vi "getAllChannelNames.vi"(8 "error in (no error)":errorcluster, 11 "ChannelArray in":refnum<class "ChannelArray.lvclass">) -> (0 "error out":errorcluster, 2 "channelNames":string[](array[string]), 3 "ChannelArray out":refnum<class "ChannelArray.lvclass">)   [LabVIEW 2009, in "Tools.lvlib" / "DatabaseHelpers.lvlib" / "ChannelArray.lvclass"]
uses:
  ChannelArray.lvclass
  ChannelArray.lvclass/ChannelArray.ctl
  Channel/Channel.lvclass
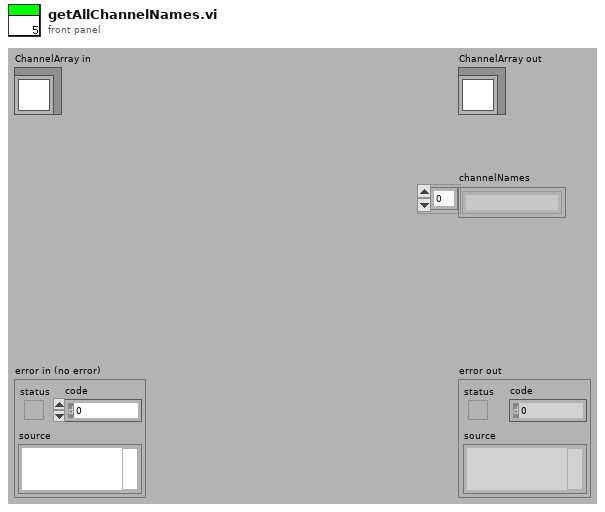
[diagram p1: front panel]
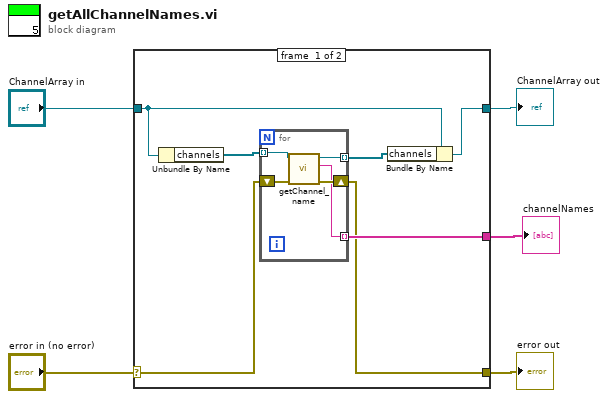
[diagram p0: block diagram]
diagram:
  n1 = case shown="No Error" "error in (no error)" {
    selector: "error in (no error)" -> [w11 w19]
    tunnel: [w6 w19] -> w4
    tunnel: [w8 w18] -> w2
    tunnel: "ChannelArray in" -> [w9 w18]
    tunnel: [w10 _] -> w1
    frame #0 {
      n2 = Unbundle By Name(w9) -> ("channels"=w12:refnum<class "Channel.lvclass">[])
      n3 = for {
        tunnel: w12 -> [w17] mode=indexing
        shift-right: [w15] -> w6
        shift-left: w11 -> [w16]
        tunnel: [w14] -> w7 mode=indexing
        tunnel: [w13] -> w10 mode=indexing
        n4 = call "getChannel_name.vi"("error in (no error)"=w16, "Channel.lvclass in"=w17) -> ("error out"=w15:errorcluster, "channel_name"=w13:string, "Channel.lvclass out"=w14:refnum<class "Channel.lvclass">)  [unwired: 7 in]
      }
      n5 = Bundle By Name(cluster=w9, "channels"=w7) -> (w8:refnum<class "ChannelArray.lvclass">)
    }
    frame #1 {
    }
  }
  "error out" <- w4
  "ChannelArray out" <- w2
  "channelNames" <- w1
